vi "PathPlanner_PathSegment_FindConstraintZone.vi"(9 "T":dbl, 11 "Zones":T1[](array[typedef])) -> (1 "IsPresent":bool, 3 "Returned Zone":T1)   [LabVIEW 2019, in "PathPlanner24.lvlib"]
doc: "Find a constraints zone within this path segment.\n\nInputs: \n - PathSegment - cluster - Data defining path segment\n - Zones - array - List of constraint zones to search.\n\nOutputs:\n - ReturnedZone - cluster - Found constraints zone definition.\n - IsPresent - boolean - TRUE if a constraints zone was found."
uses:
  PathPlanner24.lvlib
  TypeDef/PathPlannerConstraintsZone.ctl
  TypeDef/PathPlannerPathConstraints.ctl
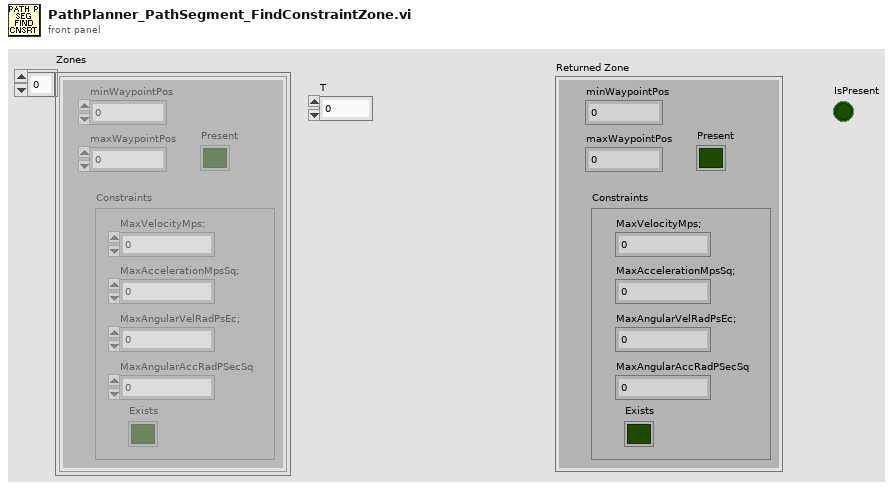
[diagram p1: front panel]
types:
  T1 = typedef "PathPlanner24.lvlib/PathPlannerConstraintsZone.ctl" = cluster{"minWaypointPos":dbl, "maxWaypointPos":dbl, "Constraints":T2, "Present":bool}
  T2 = typedef "PathPlanner24.lvlib/PathPlannerPathConstraints.ctl" = cluster{"MaxVelocityMps;":dbl, "MaxAccelerationMpsSq;":dbl, "MaxAngularVelRadPsEc;":dbl, "MaxAngularAccRadPSecSq":dbl, "Exists":bool}
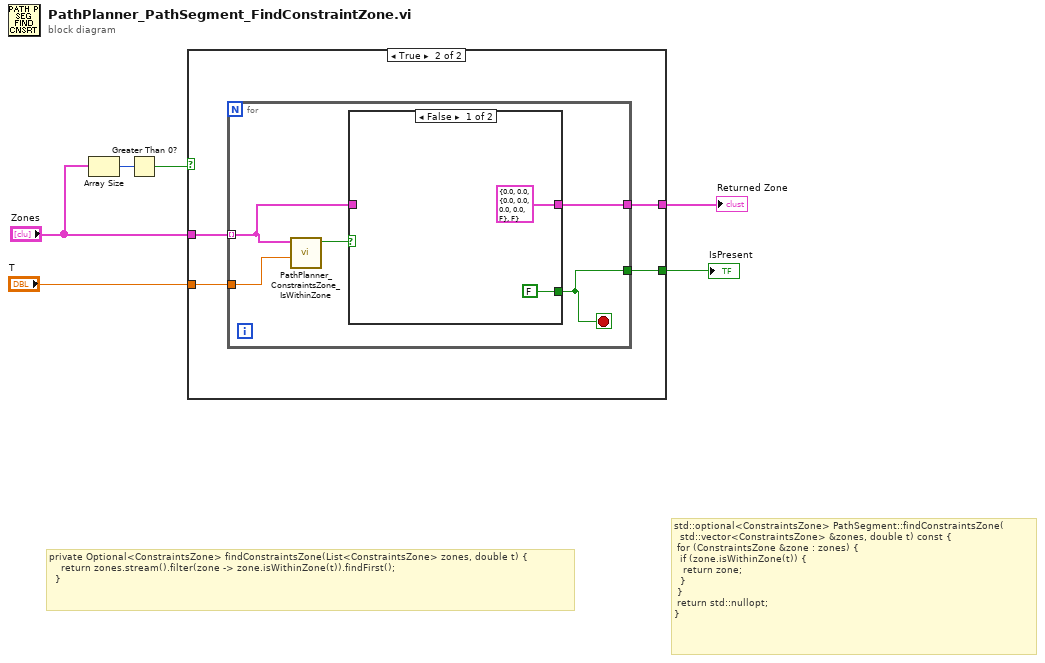
[diagram p0: block diagram]
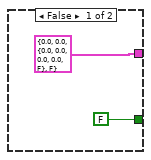
[diagram p2: hidden frame]
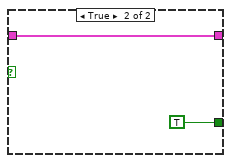
[diagram p3: hidden frame]
diagram:
  # "std::optional<ConstraintsZone> PathSegment::findConstraintsZone(\n\t\tstd::vector<ConstraintsZone> &zones, double t) const {\n\tfor (ConstraintsZone &zone : zones) {\n\t\tif (zone.isWithinZone(t)) {\n\t\t\treturn zone;\n\t\t}\n\t}\n\treturn std::nullopt;\n}"
  # "private Optional<ConstraintsZone> findConstraintsZone(List<ConstraintsZone> zones, double t) {\n    return zones.stream().filter(zone -> zone.isWithinZone(t)).findFirst();\n  }"
  n1 = Array Size(array="Zones") -> (size(s)=w2:i32)
  n2 = Greater Than 0?(x=w2) -> (x > 0?=w1:bool)
  n3 = case shown="True" w1 {
    tunnel: "T" -> [_ w12]
    tunnel: "Zones" -> [_ w11]
    tunnel: [T1 {"minWaypointPos"=0.0, "maxWaypointPos"=0.0, "Constraints"={"MaxVelocityMps;"=0.0, "MaxAccelerationMpsSq;"=0.0, "MaxAngularVelRadPsEc;"=0.0, "MaxAngularAccRadPSecSq"=0.0, "Exists"=FALSE}, "Present"=FALSE} ("ConstraintsZone") w10] -> w5
    tunnel: [FALSE w9] -> w4
    frame False {
    }
    frame True {
      n4 = for {
        tunnel: w12 -> [w17]
        tunnel: w11 -> [w15] mode=indexing
        tunnel: [w14] -> w10
        tunnel: [w13] -> w9
        stop <- w13 stop-if-true
        n5 = call "PathPlanner_ConstraintsZone_IsWithinZone.vi"("T"=w17, "ConstraintsZone"=w15) -> ("WithinZone"=w16:bool)  [unwired: 9 in]
        n6 = case shown="False" w16 {
          tunnel: w15 -> [_ w20]
          tunnel: [T1 {"minWaypointPos"=0.0, "maxWaypointPos"=0.0, "Constraints"={"MaxVelocityMps;"=0.0, "MaxAccelerationMpsSq;"=0.0, "MaxAngularVelRadPsEc;"=0.0, "MaxAngularAccRadPSecSq"=0.0, "Exists"=FALSE}, "Present"=FALSE} ("ConstraintsZone") w20] -> w14
          tunnel: [FALSE TRUE] -> w13
          frame False {
          }
          frame True {
          }
        }
      }
    }
  }
  "Returned Zone" <- w5
  "IsPresent" <- w4
